vi "Autopatch.vi"() -> ()   [LabVIEW 2018]
uses:
  <vilib>/userdefined/High Color/IMAQdx.ctl
  <vilib>/DAQmx/write.llb/DAQmx Write (Analog DBL 1Chan 1Samp).vi
  <vilib>/DAQmx/write.llb/DAQmx Write (Analog Wfm 1Chan NSamp).vi
  <vilib>/DAQmx/read.llb/DAQmx Read (Analog Wfm 1Chan NSamp).vi
  <vilib>/Analysis/baseanly.llb/Mean (DBL).vi
  <vilib>/DAQmx/create/channels.llb/DAQmx Create Channel (AO-Voltage-Basic).vi
  <vilib>/DAQmx/miscellaneous.llb/DAQmx Fill In Error Info.vi
  <vilib>/DAQmx/create/channels.llb/DAQmx Create Channel (AI-Voltage-Basic).vi
  <vilib>/DAQmx/configure/timing.llb/DAQmx Timing (Sample Clock).vi
  <vilib>/DAQmx/configure/trigger.llb/DAQmx Start Trigger (Digital Edge).vi
  <vilib>/Waveform/WDTOps.llb/WDT Waveform Duration DBL.vi
  <vilib>/addons/control/pid/pid.llb/PID (DBL).vi
  <vilib>/vision/driver/NI_Vision_Acquisition_Software.lvlib
  <vilib>/addons/control/pid/NI_PID_pid.lvlib
  <vilib>/vision/NI_Vision_Development_Module.lvlib
  <vilib>/measure/NI_MABase.lvlib
  <vilib>/Analysis/NI_AALBase.lvlib
  <resource>/objmgr/daqmx.rc
panel:
  in  "下降步伐/um":dbl=1.0
  out "封接负压增幅":dbl
  out "气压波形图表":cluster{dbl, "低负":dbl}(graph)
  in  "case":dbl
  in  "低负开关":bool
  in  "低正开关":bool
  in  "大气压":bool
  in  "高负开关":bool
  in  "高正开关":bool
  in  "低负":sgl(knob)=-0.22290154
  in  "高负":sgl(knob)=-1.1416342
  in  "低正":sgl(knob)=0.7104824 scale=0.0..2.0
  in  "高正":sgl(knob)=15.0 scale=0.0..15.0
  out "给定值":dbl
  out "测量值":dbl
  out "错误输出 2":errorcluster caption="错误输出"
  in  "DevIndex":i32
  in  "采样率":u32=255
  out "循环时间":u32
  out "！":bool
  in  "自动破膜":bool
  in  "自动封接":bool
  in  "入液阻值校准":bool
  in  "阻值数组":dbl[](array[numeric])
  in  "针尖模板匹配":bool
  in  "自动接触":bool
  in  "文件路径（使用对话框）":path=path "E:/膜片/实验/数据"
  in  "保存图像和数据":bool
  in  "控制箱刺激/放大器刺激":bool=TRUE
  in  "frequency":dbl=20.0
  in  "Averaging":i32=3
  in  "amplitude":dbl=0.01
  in  "下拉列表":u16(ring) items=["Voltage Clamp", "Current Clamp"]
  in  "Holding Voltage":dbl
  out "Resistance":dbl
  out "电阻值2":dbl
  out "阻值波形图表":dbl(graph)
  out "校准的入液阻值":dbl
  in  "Session In":T1="cam1"
  out "目标坐标":i32[](array[numeric])
  in  "Number of Erosion":i32=10
  in  "Operation":T2(ring)=enum."Dilate"
  out "布尔":bool
  in  "自动聚焦":bool
  in  "细调焦":bool
  in  "Range":cluster{"Lower value":sgl, "Upper value":sgl}={"Lower value"=0.0, "Upper value"=86.0} {"Upper value" format="%.2f"; "Lower value" format="%.2f"}
  in  "Minimum Match Score":sgl=500.0 min=0 max=1000 format="%.2f"
  out "Number of Matches":i32
  in  "自动移动":bool
  out "Image":T3(plugin-control)
  in  "停止":bool
  out "错误输出":errorcluster
  in  "基路径":path=path "E:/膜片/膜片钳/程序/CCD/模板40倍.jpg"
  out "针尖坐标":sgl[](array[numeric])
  out "电信号波形图":waveform(dbl)(graph)
  out "Negative Peak":dbl
  out "mean":dbl caption="均值" format="%0.2f"
  in  "Minimum Contrast":i32 min=0 max=255 step=1
  in  "Number of Matches Requested":i32=1 min=1
  out "Matches 2":T4(array[cluster]) {"Bounding Box"."y" format="%.2f"; "Bounding Box"."x" format="%.2f"; "Position"."y" format="%.2f"; "Position"."x" format="%.2f"; "Score" format="%.2f"; "Scale" format="%.2f"; "Angle" format="%.2f"}
  in  "Match Mode":u16(ring) items=["Shift Invariant", "Rotation Invariant"]
  out "二值化":T3(plugin-control)
  in  "PID gains":T5={"proportional gain (Kc)"=-0.5, "integral time (Ti, min)"=0.0, "derivative time (Td, min)"=0.0} caption="PID增益" {"derivative time (Td, min)" format="%.3f"; "integral time (Ti, min)" format="%.3f"; "proportional gain (Kc)" format="%.3f"}
  in  "PID gains 2":T5={"proportional gain (Kc)"=0.5, "integral time (Ti, min)"=0.0, "derivative time (Td, min)"=0.0} caption="PID增益" {"derivative time (Td, min)" format="%.3f"; "integral time (Ti, min)" format="%.3f"; "proportional gain (Kc)" format="%.3f"}
  out "评价函数":dbl(graph)
  in  "聚焦值数组":dbl[](array[numeric])
  out "数组最大值":dbl
  out "调焦值2":dbl
  out "数值 3":dbl
  out "数值 4":dbl
  out "变量":dbl
  out "x+y 2":i16
  out "Particle Reports (Pixels)":T6(array[cluster]) {"Orientation" format="%.2f"; "Dimensions"."Height" format="%.2f"; "Dimensions"."Width" format="%.2f"; "Center of Mass"."Y" format="%.2f"; "Center of Mass"."X" format="%.2f"; "Bounding Rect"."Bottom" format="%.2f"; "Bounding Rect"."Right" format="%.2f"; "Bounding Rect"."Top" format="%.2f"; "Bounding Rect"."Left" format="%.2f"; "Number of Holes" format="%.2f"; "Area" format="%.2f"}
  out "Right":dbl
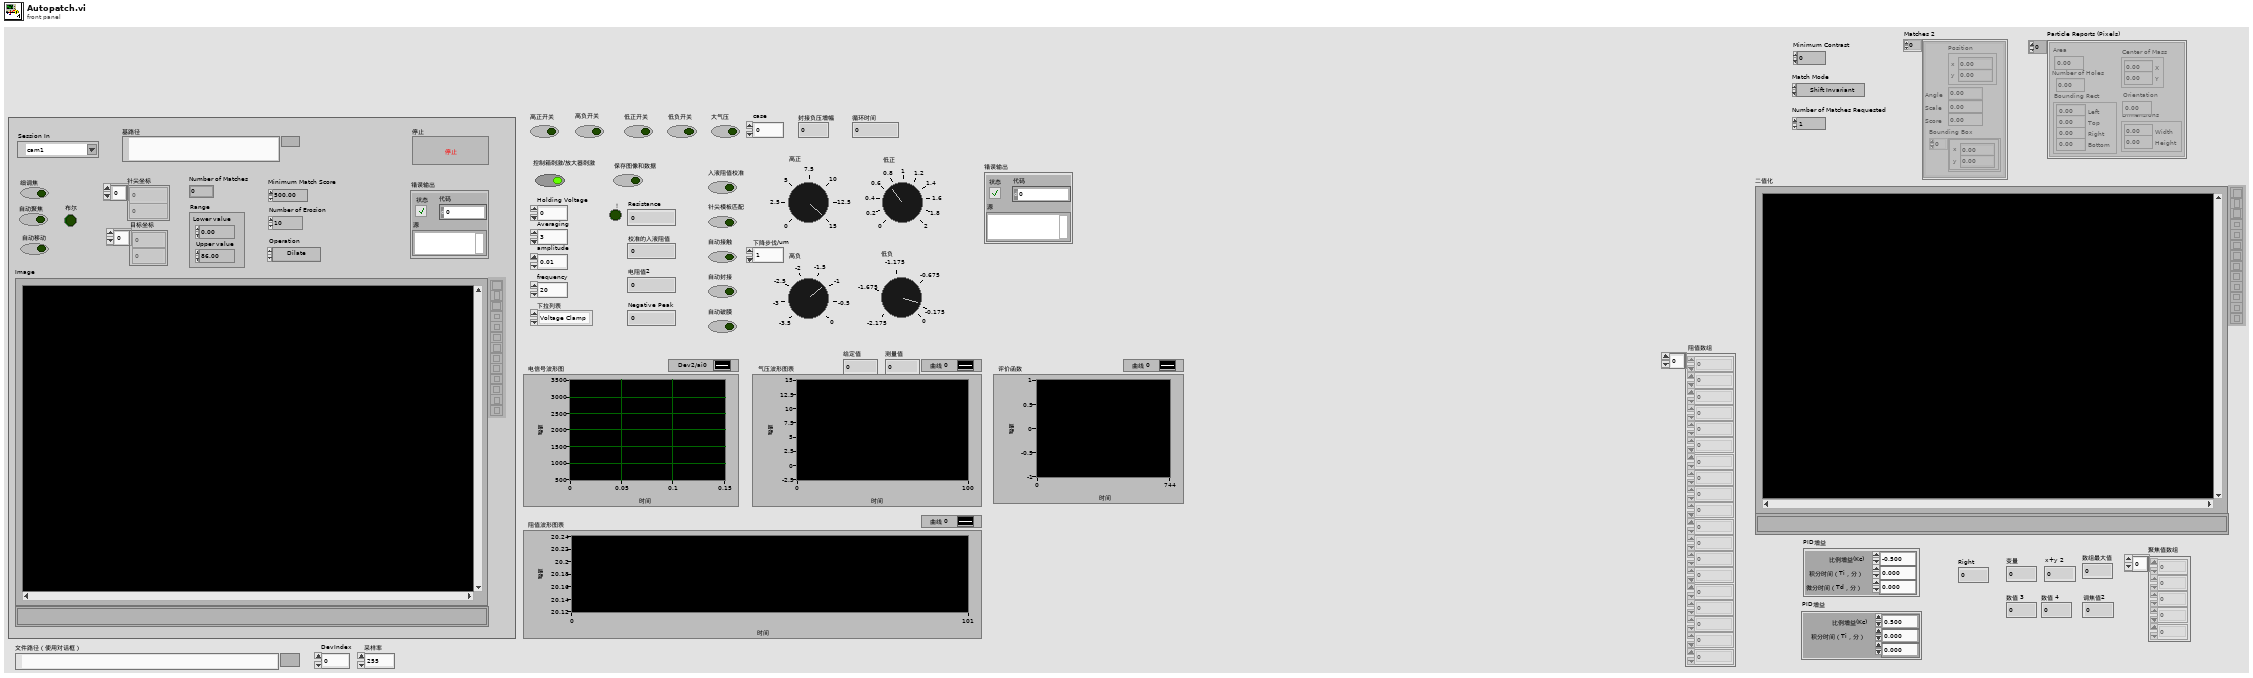
[diagram p1: front panel]
types:
  T1 = typedef "IMAQdx.ctl" = refnum<k21>
  T2 = enum32{"AutoM", "Close", "Dilate", "Erode", "Gradient", "Gradient out", "Gradient in", "Hit miss", "Open", "PClose", "POpen", "Thick", "Thin"}
  T3 = typedef "IMAQ Image.ctl" = refnum<image>
  T4 = cluster{"Position":cluster{"x":sgl, "y":sgl}, "Angle":sgl, "Scale":sgl, "Score":sgl, "Bounding Box":cluster{"x":sgl, "y":sgl}[]}[]
  T5 = cluster{"proportional gain (Kc)":dbl, "integral time (Ti, min)":dbl, "derivative time (Td, min)":dbl}
  T6 = cluster{"Area":dbl, "Number of Holes":dbl, "Bounding Rect":cluster{"Left":dbl, "Top":dbl, "Right":dbl, "Bottom":dbl}, "Center of Mass":cluster{"X":dbl, "Y":dbl}, "Orientation":dbl, "Dimensions":cluster{"Width":dbl, "Height":dbl}}[]
  T7 = typedef "Image Type" = u32
  T8 = enum16{"open", "replace", "create", "open or create", "replace or create", "replace or create with confirmation"}
  T9 = cluster{"Averaging":i32, "frequency":dbl, "amplitude":dbl, "Proportion":dbl, "Fs":dbl}
  T10 = enum16{"Sine Wave", "Triangle Wave", "Square Wave", "Sawtooth Wave"}
  T11 = cluster{"Position":cluster{"x":sgl, "y":sgl}, "Angle":sgl, "Scale":sgl, "Score":sgl, "Bounding Box":cluster{"x":sgl, "y":sgl}[]}
  T12 = cluster{"Global Rectangle":i32[], "Contours":cluster{"Contour Type":u32, "ROI Type":u32, "Points":i32[]}[]}
  T13 = cluster{"Area":dbl, "Number of Holes":dbl, "Bounding Rect":cluster{"Left":dbl, "Top":dbl, "Right":dbl, "Bottom":dbl}, "Center of Mass":cluster{"X":dbl, "Y":dbl}, "Orientation":dbl, "Dimensions":cluster{"Width":dbl, "Height":dbl}}
  T14 = cluster{"Left":dbl, "Top":dbl, "Right":dbl, "Bottom":dbl}
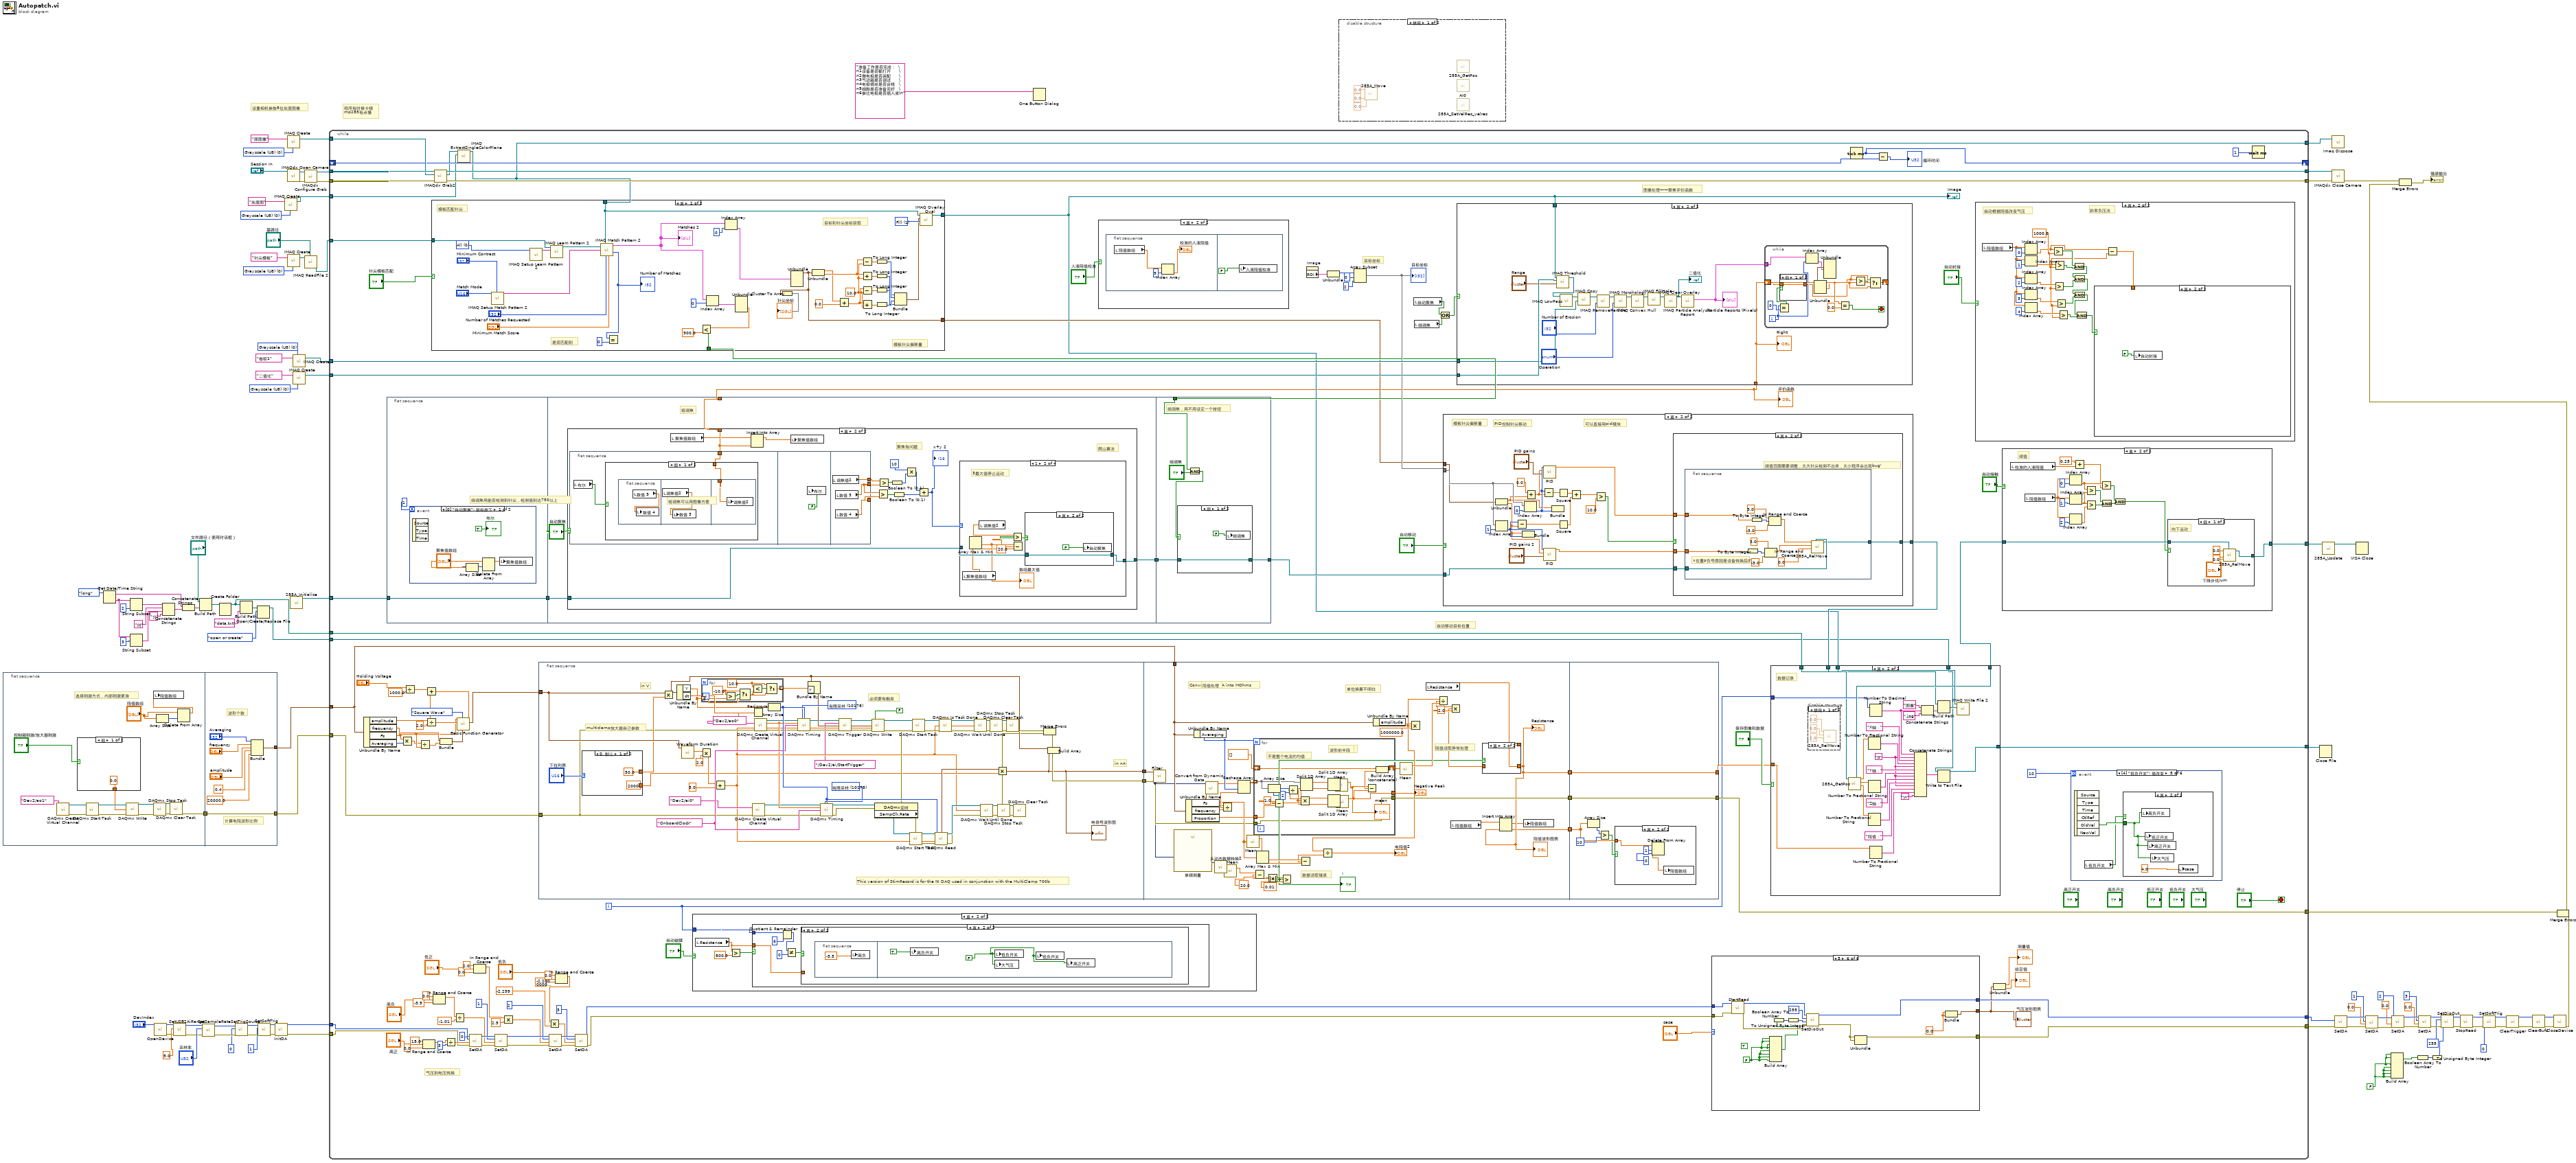
[diagram p0: block diagram]
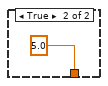
[diagram p2: hidden frame]
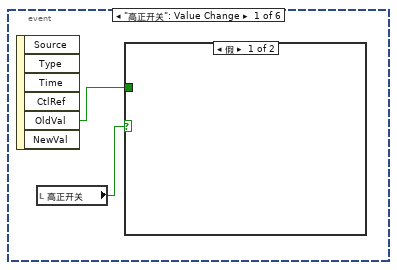
[diagram p4: hidden frame]
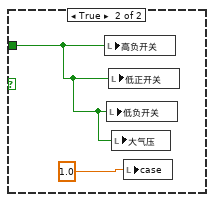
[diagram p5: hidden frame]
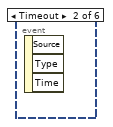
[diagram p6: hidden frame]
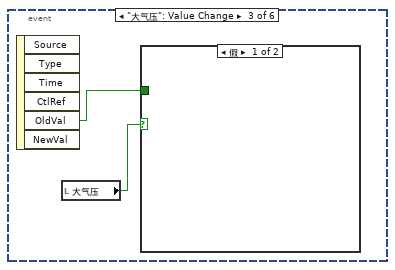
[diagram p7: hidden frame]
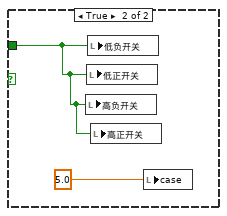
[diagram p8: hidden frame]
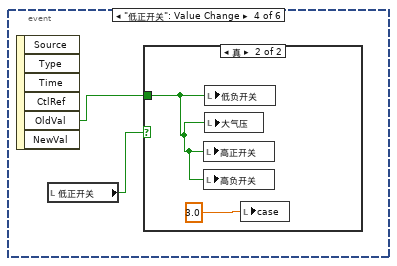
[diagram p9: hidden frame]
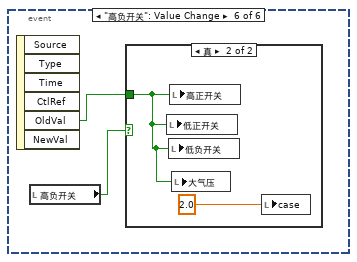
[diagram p12: hidden frame]
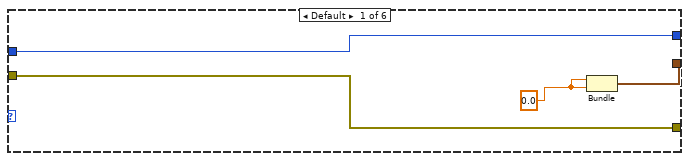
[diagram p14: hidden frame]
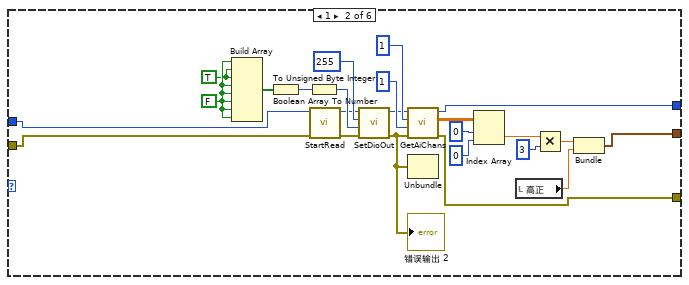
[diagram p15: hidden frame]
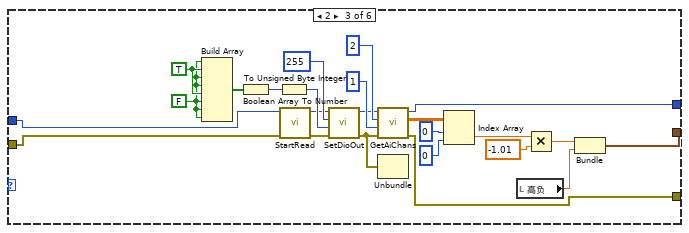
[diagram p16: hidden frame]
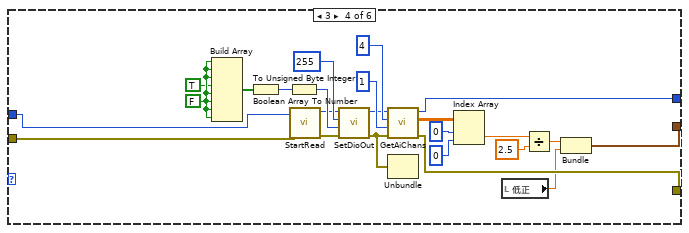
[diagram p17: hidden frame]
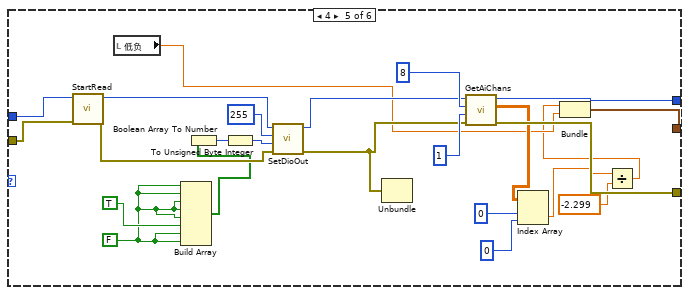
[diagram p18: hidden frame]
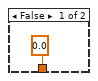
[diagram p19: hidden frame]
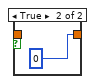
[diagram p20: hidden frame]
diagram:
  w12 = FALSE
  w55 = T7 0 items=["Grayscale (U8)", "Grayscale (I16)", "Grayscale (SGL)", "Complex (CSG)", "RGB (U32)", "HSL (U32)", "RGB (U64)", "Grayscale (U16)"] ("Image Type")
  w57 = T7 0 items=["Grayscale (U8)", "Grayscale (I16)", "Grayscale (SGL)", "Complex (CSG)", "RGB (U32)", "HSL (U32)", "RGB (U64)", "Grayscale (U16)"] ("Image Type")
  w58 = T7 0 items=["Grayscale (U8)", "Grayscale (I16)", "Grayscale (SGL)", "Complex (CSG)", "RGB (U32)", "HSL (U32)", "RGB (U64)", "Grayscale (U16)"] ("Image Type")
  w59 = T7 0 items=["Grayscale (U8)", "Grayscale (I16)", "Grayscale (SGL)", "Complex (CSG)", "RGB (U32)", "HSL (U32)", "RGB (U64)", "Grayscale (U16)"] ("Image Type")
  w60 = T7 0 items=["Grayscale (U8)", "Grayscale (I16)", "Grayscale (SGL)", "Complex (CSG)", "RGB (U32)", "HSL (U32)", "RGB (U64)", "Grayscale (U16)"] ("Image Type")
  # "程序有时候卡顿\nmp285有点慢"
  # "设置相机参数8位灰度图像"
  n1 = flat-sequence {
    tunnel: [w109] -> w62
    tunnel: [w124] -> w81
    tunnel: [w123] -> w61
    tunnel: w62 -> [w123]
    frame #0 {
      # "选择刺激方式，内部刺激更准"
      n2 = call-poly <vilib>:"DAQmx Create Virtual Channel.vi"("physical channels"=tag "Dev2/ao1") -> ("task out"=w116:refnum<k21>, "error out"=w115:errorcluster)  [unwired: 13 in]
      n3 = case shown="假" "控制箱刺激/放大器刺激" {
        tunnel: [0.0 ("data") 5.0 ("data")] -> w112
        frame False {
        }
        frame True {
        }
      }
      n4 = call <vilib>:"DAQmx Start Task.vi"("task/channels in"=w116, "error in"=w115) -> ("task out"=w117:refnum<k21>, "error out"=w118:errorcluster)  [unwired: 12 in]
      n5 = call-poly <vilib>:"DAQmx Write.vi"("task/channels in"=w117, "data"=w112, "error in"=w118) -> ("task out"=w119:refnum<k21>, "error out"=w120:errorcluster)  [unwired: 10 in, 1 out]
      n6 = call <vilib>:"DAQmx Stop Task.vi"("task/channels in"=w119, "error in"=w120) -> ("task out"=w113:refnum<k21>, "error out"=w114:errorcluster)  [unwired: 12 in]
      n7 = Array Size(array="阻值数组") -> (size(s)=w108:i32)
      n8 = call <vilib>:"DAQmx Clear Task.vi"("task in"=w113, "error in"=w114) -> ("error out"=w109:errorcluster)  [unwired: 13 in]
      n9 = Delete From Array(array="阻值数组", length=w108) -> (array with subset deleted=w106:dbl[])  [unwired: 1 in, 1 out]
      n10 = local write "阻值数组"(w106) -> ()
    }
    frame #1 {
      # "波形个数"
      # "计算电阻波形比例"
      n11 = Bundle("Averaging"="Averaging", "frequency"="frequency", "amplitude"="amplitude", "Proportion"=0.4, "Fs"=20000.0) -> (w124:T9)  [unwired: 1 in]
    }
  }
  n12 = Get Date/Time String(date format (0)=enum16{"short", "long", "abbreviated"}."long" ("日期格式(0)")) -> (date string=w77:string, time string=w73:string)  [unwired: 2 in]
  n13 = String Subset(string=w73, length (rest)=2 ("长度（剩余）")) -> (substring=w71:string)  [unwired: 1 in]
  n14 = String Subset(string=w73, offset (0)=3 ("偏移量(0)")) -> (substring=w69:string)  [unwired: 1 in]
  n15 = call "OpenDevice.vi"("DevIndex"="DevIndex") -> ("错误输出"=w39:errorcluster, "DevIndex Output"=w37:i32)  [unwired: 9 in]
  n16 = Concatenate Strings(w71, "时" ("字符串"), w69, "分" ("字符串")) -> (w70:string)
  n17 = call "SetUSB2AiRange.vi"("错误输入（无错误）"=w39, "Range"=sgl 5.0, "DevIndex"=w37) -> ("错误输出"=w48:errorcluster, "DevIndex Output"=w46:i32)  [unwired: 7 in]
  n18 = Concatenate Strings(w77, w70) -> (w66:string)
  n19 = Build Path(base path="文件路径（使用对话框）", name or relative path=w66) -> (appended path=w67:path)
  n20 = call "SetSampleRate.vi"("错误输入（无错误）"=w48, "SampleRate"="采样率", "DevIndex"=w46) -> ("错误输出"=w49:errorcluster, "DevIndex Output"=w47:i32)  [unwired: 7 in]
  n21 = Create Folder(path (use dialog)=w67) -> (created path=w65:path)  [unwired: 2 in, 2 out]
  n22 = call "SetTrigSource.vi"("错误输入（无错误）"=w49, "TrigSource"=u8 0, "DevIndex"=w47) -> ("错误输出"=w44:errorcluster, "DevIndex Output"=w43:i32)  [unwired: 7 in]
  n23 = Build Path(base path=w65, name or relative path="data.txt" ("字符串")) -> (appended path=w56:path)
  n24 = Open/Create/Replace File(file path (use dialog)=w56, operation (0:open)=T8."open or create" ("操作(0:open)")) -> (refnum out=w52:refnum<file>)  [unwired: 4 in, 2 out]
  n25 = call "SetSoftTrig.vi"("错误输入（无错误）"=w44, "Trig"=u8 1, "DevIndex"=w43) -> ("错误输出"=w40:errorcluster, "DevIndex Output"=w38:i32)  [unwired: 7 in]
  n26 = call "InitDA.vi"("错误输入（无错误）"=w40, "DevIndex"=w38) -> ("错误输出"=w34:errorcluster, "DevIndex Output"=w35:i32)  [unwired: 8 in]
  n27 = call "IMAQ Create"("Image Name"="灰度图", "Image Type"=w55) -> ("New Image"=w53:T3)  [unwired: 3 in, 1 out]
  n28 = call "IMAQ Create"("Image Name"="原图像", "Image Type"=w60) -> ("New Image"=w95:T3)  [unwired: 3 in, 1 out]
  n29 = call <vilib>:"IMAQdx Open Camera.vi"("Session In"="Session In") -> ("error out"=w104:errorcluster, "Session Out"=w103:T1)  [unwired: 9 in]
  n30 = call "IMAQ Create"("Image Name"="针尖模板", "Image Type"=w59) -> ("New Image"=w90:T3)  [unwired: 3 in, 1 out]
  n31 = call "285A_Initialize.vi"() -> ("VISA资源名称输出"=w82:refnum<visa-resource-name>)  [unwired: 10 in, 1 out]
  n32 = call "IMAQ Create"("Image Name"="卷积1", "Image Type"=w58) -> ("New Image"=w87:T3)  [unwired: 3 in, 1 out]
  n33 = call "IMAQ Create"("Image Name"="二值化", "Image Type"=w57) -> ("New Image"=w86:T3)  [unwired: 3 in, 1 out]
  n34 = call <vilib>:"IMAQdx Configure Grab.vi"("error in"=w104, "Session In"=w103) -> ("error out"=w102:errorcluster, "Session Out"=w101:T1)  [unwired: 8 in]
  n35 = call "IMAQ ReadFile 2"("File Path"="基路径", "Image"=w90) -> ("Image Out"=w89:T3)  [unwired: 5 in, 4 out]
  n36 = while {
    tunnel: w101 -> [w244]
    tunnel: w95 -> [w243]
    tunnel: [w242] -> w96
    tunnel: [w185] -> w97
    tunnel: w102 -> [w240]
    tunnel: [w239] -> w98
    tunnel: w89 -> [w238]
    tunnel: w87 -> [w233]
    tunnel: w86 -> [w237]
    tunnel: w82 -> [w234]
    tunnel: [w193] -> w84
    tunnel: w81 -> [w148]
    tunnel: w61 -> [w213]
    tunnel: [w198] -> w79
    tunnel: w65 -> [w207]
    shift-right: [w188] -> _
    shift-left: _ -> [w189]
    tunnel: w53 -> [w184]
    tunnel: w52 -> [w179]
    tunnel: [w178] -> w51
    tunnel: w35 -> [w160]
    tunnel: w34 -> [w159]
    tunnel: [w153] -> w3
    tunnel: [w156] -> w2
    i -> [w147]
    stop <- "停止" stop-if-true
    # "气压到电压转换"
    # "目标坐标"
    # "图像处理——聚焦评价函数"
    # "自动移动目标位置"
    # "粗调焦可以用图像方差"
    # "细调焦用能否检测到针尖，检测值到达750以上"
    n37 = Unbundle By Name(w148) -> ("amplitude"=w218:dbl, "frequency"=w217:dbl, "Fs"=w219:dbl, "Averaging"=w220:i32)
    n38 = flat-sequence {
      tunnel: w234 -> [w716]
      tunnel: [w716] -> w236
      tunnel: w236 -> [w723]
      tunnel: [w722] -> w235
      tunnel: w180 -> [w721]
      tunnel: [w803] -> w232
      tunnel: w235 -> [w804]
      tunnel: w229 -> [w801]
      frame #0 {
        n39 = event shown="[0] \"自动聚焦\": 鼠标按下" {
          selector: _ -> [_ _]
          dyn-events: _ -> [_ _]
          timeout: 1 -> [_ _]
          event "自动聚焦": Mouse Down {
            n40 = event-data() -> ()  [unwired: 1 in, 3 out]
            n41 = Array Size(array="聚焦值数组") -> (size(s)=w717:i32)
            n42 = Delete From Array(array="聚焦值数组", length=w717) -> (array with subset deleted=w718:dbl[])  [unwired: 1 in, 1 out]
            n43 = local write "聚焦值数组"(w718) -> ()
            "布尔" <- TRUE
          }
          event Timeout {
            n44 = event-data() -> ()  [unwired: 1 in, 3 out]
          }
        }
      }
      frame #1 {
        # "粗调焦"
        n45 = case shown="真" "自动聚焦" {
          tunnel: w723 -> [w725 w734]
          tunnel: [w725 w733] -> w722
          tunnel: w721 -> [_ w732]
          frame False {
          }
          frame True {
            # "聚焦有问题"
            # "爬山算法"
            n46 = flat-sequence {
              tunnel: w732 -> [w742]
              tunnel: [w752] -> w740
              tunnel: [w751] -> w738
              tunnel: [w750] -> w739
              frame #0 {
                n47 = local read "布尔"() -> (w741:bool)
                n48 = case shown="假" w741 {
                  tunnel: w742 -> [w743 w747]
                  frame False {
                    n49 = flat-sequence {
                      tunnel: w743 -> [w746]
                      frame #0 {
                        n50 = local read "数值 3"() -> (w744:dbl)
                        n51 = local write "数值 4"(w744) -> ()
                      }
                      frame #1 {
                        n52 = local read "调焦值2"() -> (w745:dbl)
                        n53 = local write "数值 3"(w745) -> ()
                      }
                      frame #2 {
                        n54 = local write "调焦值2"(w746) -> ()
                      }
                    }
                  }
                  frame True {
                    # "第一次赋值"
                    "调焦值2" <- w747
                    "数值 3" <- w747
                    "数值 4" <- w747
                    "变量" <- 1
                  }
                }
              }
              frame #1 {
                n55 = local write "布尔"(FALSE) -> ()
              }
              frame #2 {
                n56 = local read "调焦值2"() -> (w752:dbl)
                n57 = local read "数值 3"() -> (w751:dbl)
                n58 = local read "数值 4"() -> (w750:dbl)
              }
            }
            n59 = local read "聚焦值数组"() -> (w731:dbl[])
            n60 = Insert Into Array(array=w731, new element=w732) -> (w730:dbl[])  [unwired: 1 in]
            n61 = local write "聚焦值数组"(w730) -> ()
            n62 = Greater?(x=w738, y=w739) -> (0:w737:bool)
            n63 = Greater?(x=w740, y=w738) -> (0:w729:bool)
            n64 = Boolean To (0,1)(Boolean=w729) -> (0, 1=w728:i16)
            n65 = Boolean To (0,1)(Boolean=w737) -> (0, 1=w727:i16)
            n66 = Multiply(x=i16 10, y=w728) -> (x*y=w735:i16)
            n67 = Add(x=w735, y=w727) -> (x+y=w726:i16)
            "x+y 2" <- w726
            n68 = case shown="1" w726 {
              tunnel: [w759 w764 w778 w786] -> w733
              tunnel: w734 -> [w757 w765 w777 w787]
              frame 11, Default {
                # "1往上运动"
                n69 = local read "变量"() -> (w753:dbl)
                n70 = Multiply(x=10.0 ("Z 2"), y=w753) -> (x*y=w754:dbl)
                n71 = call "285A_RelMove.vi"("VISA资源名称"=w757, "Z 2"=w754, "Y 2"=0.0, "X 2"=0.0) -> ("VISA resource name out 2"=w759:refnum<visa-resource-name>)  [unwired: 2 in, 5 out]
              }
              frame 1 {
                # "3最大值停止运动"
                n72 = local read "聚焦值数组"() -> (w760:dbl[])
                n73 = Array Max & Min(array=w760) -> (max value=w763:dbl)  [unwired: 3 out]
                "数组最大值" <- w763
                n74 = local read "调焦值2"() -> (w767:dbl)
                n75 = Subtract(x=w763, y=20.0) -> (x-y=w761:dbl)
                n76 = Greater?(x=w767, y=w761) -> (0:w766:bool)
                n77 = case shown="真" w766 {
                  tunnel: [w768 w775] -> w764
                  tunnel: w765 -> [w773 w775]
                  frame False {
                    n78 = local read "变量"() -> (w770:dbl)
                    n79 = Multiply(x=20.0 ("Z 2"), y=w770) -> (x*y=w771:dbl)
                    n80 = call "285A_RelMove.vi"("VISA资源名称"=w773, "Z 2"=w771, "Y 2"=0.0, "X 2"=0.0) -> ("VISA resource name out 2"=w768:refnum<visa-resource-name>)  [unwired: 2 in, 5 out]
                  }
                  frame True {
                    n81 = local write "自动聚焦"(FALSE) -> ()
                  }
                }
              }
              frame 10 {
                # "4继续向上运动"
                n82 = flat-sequence {
                  tunnel: [w783] -> w778
                  tunnel: w777 -> [w782]
                  frame #0 {
                    n83 = local read "变量"() -> (w779:dbl)
                    n84 = Multiply(x=10.0 ("Z 2"), y=w779) -> (x*y=w780:dbl)
                    n85 = call "285A_RelMove.vi"("VISA资源名称"=w782, "Z 2"=w780, "Y 2"=0.0, "X 2"=0.0) -> ("VISA resource name out 2"=w783:refnum<visa-resource-name>)  [unwired: 2 in, 5 out]
                  }
                }
              }
              frame 0 {
                # "2向回运动"
                n86 = flat-sequence {
                  tunnel: w787 -> [w792]
                  tunnel: [w792] -> w788
                  tunnel: [w797] -> w786
                  tunnel: w788 -> [w796]
                  frame #0 {
                    n87 = local read "变量"() -> (w791:dbl)
                    n88 = Multiply(x=w791, y=-1) -> (x*y=w789:dbl)
                    n89 = local write "变量"(w789) -> ()
                  }
                  frame #1 {
                    n90 = local read "变量"() -> (w793:dbl)
                    n91 = Multiply(x=10.0 ("Z 2"), y=w793) -> (x*y=w794:dbl)
                    n92 = call "285A_RelMove.vi"("VISA资源名称"=w796, "Z 2"=w794, "Y 2"=0.0, "X 2"=0.0) -> ("VISA resource name out 2"=w797:refnum<visa-resource-name>)  [unwired: 2 in, 5 out]
                  }
                }
              }
            }
          }
        }
      }
      frame #2 {
        # "细调焦，用不用设定一个按钮"
        n93 = And(x=w801, y="细调焦") -> (x .and. y?=w802:bool)
        n94 = case shown="假" w802 {
          tunnel: [w806 w807] -> w803
          tunnel: w804 -> [w806 w808]
          frame False {
            n95 = local write "细调焦"(FALSE) -> ()
          }
          frame True {
            n96 = local read "变量"() -> (w810:dbl)
            n97 = Multiply(x=10.0 ("Z 2"), y=w810) -> (x*y=w809:dbl)
            n98 = call "285A_RelMove.vi"("VISA资源名称"=w808, "Z 2"=w809, "Y 2"=0.0, "X 2"=0.0) -> ("VISA resource name out 2"=w807:refnum<visa-resource-name>)  [unwired: 2 in, 5 out]
          }
        }
      }
    }
    n99 = Multiply(x=w219, y=w220) -> (x*y=w215:dbl)
    n100 = Divide(x="Holding Voltage", y=1000.0) -> (x/y=w224:dbl)
    n101 = Divide(x=w215, y=w217) -> (x/y=w216:dbl)
    n102 = In Range and Coerce(upper limit=sgl 15.0 ("上限"), x="高正", lower limit=sgl 0.0 ("下限")) -> (coerced(x)=w132:sgl)  [unwired: 1 out]
    n103 = Divide(x=w218, y=2.0) -> (x/y=w223:dbl)
    n104 = Add(x=w224, y=w223) -> (x+y=w222:dbl)
    n105 = In Range and Coerce(upper limit=sgl 0.0 ("上限"), x="高负", lower limit=sgl -3.5 ("下限")) -> (coerced(x)=w136:sgl)  [unwired: 1 out]
    n106 = call <vilib>:"IMAQdx Grab2.vi"("error in"=w240, "Image In"=w243, "Session In"=w244) -> ("error out"=w239:errorcluster, "Image Out"=w186:T3, "Session Out"=w242:T1)  [unwired: 5 in, 1 out]
    n107 = Bundle("Fs"=w219, w216) -> (w221:cluster{"Fs":dbl, dbl})  [unwired: 1 in]
    n108 = Divide(x=w132, y=3) -> (x/y=w167:sgl)
    n109 = Divide(x=w136, y=-1.01) -> (x/y=w163:dbl)
    n110 = call <vilib>:"Basic Function Generator.vi"("offset"=w222, "sampling info"=w221, "signal type"=T10."Square Wave", "amplitude"=w223, "frequency"=w217) -> ("signal out"=w228:waveform(dbl))  [unwired: 4 in, 2 out]
    n111 = call "IMAQ ExtractSingleColorPlane"("Image Dst"=w184, "Image Src"=w186) -> ("Image Dst Out"=w185:T3)  [unwired: 8 in, 1 out]
    n112 = case shown="真" "针尖模板匹配" {
      tunnel: w238 -> [_ w519]
      tunnel: w185 -> [w479 w483]
      tunnel: [FALSE w518] -> w229
      tunnel: [w478 w486] -> w200
      tunnel: [w479 w482] -> w199
      frame False {
        w480 = 0.0 ("x")
        n113 = Bundle("x"=w480, "x"=w480) -> (w478:cluster{"x":dbl, "x":dbl})  [unwired: 1 in]
      }
      frame True {
        w485 = u32 1 items=["Frame", "Fill", "Highlight"] ("Drawing Mode (Frame)")
        w488 = 10.0 ("y")
        w512 = u16 0 items=["All", "Shift Information", "Rotation Information"] ("Learn Mode")
        # "目标和针尖坐标获取"
        # "模板针尖偏移量"
        # "是否匹配到"
        # "模板匹配针尖"
        n114 = call "IMAQ Setup Match Pattern 2"("Minimum Contrast"="Minimum Contrast", "Match Mode"="Match Mode") -> ("Match Pattern Setup Data"=w516:string)  [unwired: 8 in, 1 out]
        n115 = call "IMAQ Setup Learn Pattern 2"("Learn Mode"=w512) -> ("Learn Pattern Setup Data"=w511:string)  [unwired: 9 in, 1 out]
        n116 = call "IMAQ Learn Pattern 2"("Learn Pattern Setup Data"=w511, "Image"=w519) -> ("Template Image Out"=w508:T3)  [unwired: 8 in, 1 out]
        n117 = call "IMAQ Match Pattern 2"("Minimum Match Score"="Minimum Match Score", "Number of Matches Requested"="Number of Matches Requested", "Match Pattern Setup Data"=w516, "Template Image"=w508, "Image"=w483) -> ("Number of Matches"=w509:i32, "Matches"=w505:T4)  [unwired: 4 in, 1 out]
        "Number of Matches" <- w509
        "Matches 2" <- w505
        n118 = Equal?(x=w509, y=0) -> ()  [unwired: 1 out]
        n119 = Index Array(array=w505, index=0 ("索引")) -> (element=w503:T11)
        n120 = Index Array(array=w505, index=0 ("索引")) -> (element=w487:T11)
        n121 = Unbundle(w503) -> ("Score"=w502:sgl)  [unwired: 4 out]
        n122 = Less?(x=w502, y=sgl 900.0) -> (x < y?=w518:bool)
        n123 = Unbundle(w487) -> ("Position"=w486:cluster{"x":sgl, "y":sgl})  [unwired: 4 out]
        n124 = Cluster To Array(cluster=w486) -> (array=→"针尖坐标":sgl[])
        n125 = Unbundle(w486) -> ("x"=w497:sgl, "y"=w500:sgl)
        n126 = Add(x=w497, y=sgl 0.0) -> (x+y=w499:sgl)
        n127 = Subtract(x=w500, y=w488) -> (x-y=w491:dbl)
        n128 = Add(x=w500, y=w488) -> (x+y=w490:dbl)
        n129 = Subtract(x=w499, y=w488) -> (x-y=w489:dbl)
        n130 = Add(x=w499, y=w488) -> (x+y=w492:dbl)
        n131 = To Long Integer(number=w491) -> (32bit integer=w494:i32)
        n132 = To Long Integer(number=w490) -> (32bit integer=w495:i32)
        n133 = To Long Integer(number=w489) -> (32bit integer=w493:i32)
        n134 = To Long Integer(number=w492) -> (32bit integer=w496:i32)
        n135 = Bundle(w493, w494, w496, w495) -> (w484:cluster{i32, i32, i32, i32})  [unwired: 1 in]
        n136 = call "IMAQ Overlay Oval"("Drawing Mode (Frame)"=w485, "Bounding Rectangle"=w484, "Image"=w483) -> ("Image Out"=w482:T3)  [unwired: 7 in, 1 out]
      }
    }
    "Image" <- w199
    n137 = call "SetDA.vi"("错误输入（无错误）"=w159, "DAVolt"=w167, "DANum"=u8 0, "DevIndex"=w160) -> ("错误输出"=w176:errorcluster, "DevIndex Output"=w177:i32)  [unwired: 6 in]
    n138 = In Range and Coerce(upper limit=sgl 2.0 ("上限"), x="低正", lower limit=sgl 0.0 ("下限")) -> (coerced(x)=w140:sgl)  [unwired: 1 out]
    n139 = call "SetDA.vi"("错误输入（无错误）"=w176, "DAVolt"=w163, "DANum"=u8 1, "DevIndex"=w177) -> ("错误输出"=w175:errorcluster, "DevIndex Output"=w174:i32)  [unwired: 6 in]
    n140 = Multiply(x=w140, y=2.5) -> (x*y=w154:dbl)
    n141 = flat-sequence {
      tunnel: w228 -> [w596]
      tunnel: w213 -> [w592]
      tunnel: [w597] -> w212
      tunnel: [w581] -> w211
      tunnel: w212 -> [w665]
      tunnel: w211 -> [w666]
      tunnel: w148 -> [w667]
      tunnel: [w664] -> w197
      tunnel: [w654] -> w196
      tunnel: [w652] -> w195
      tunnel: [w709] -> w208
      tunnel: [w710] -> w198
      tunnel: w197 -> [w710]
      tunnel: w196 -> [w709]
      tunnel: w195 -> [w707]
      frame #0 {
        w626 = 10178 items=["有限采样"=10178, "连续采样"=10123, "硬件定时单点"=12522] ("sample mode")
        w627 = tag "OnboardClock" ("source")
        w619 = 10178 items=["有限采样"=10178, "连续采样"=10123, "硬件定时单点"=12522] ("sample mode")
        # "必须要有触发"
        # "This version of StimRecord is for the NI DAQ used in conjunction with the MultiClamp 700b"
        # "multiclamp放大器自己参数"
        # "in V"
        # "in nA"
        n142 = case shown="0, 默认" "下拉列表" {
          tunnel: [50.0 ("y") 2500000000.0 ("y")] -> w593
          tunnel: [2000.0 ("y") 0.1 ("y")] -> w594
          frame 0, Default {
          }
          frame 1 {
          }
        }
        n143 = Multiply(x=w596, y=w593) -> (x*y=w612:waveform(dbl))
        n144 = Unbundle By Name(w612) -> ("Y"=w580:dbl[], "dt"=w611:dbl)
        n145 = call-poly <vilib>:"Waveform Duration.vi"("waveform in"=w596) -> ("duration"=w614:dbl)  [unwired: 8 in, 2 out]
        n146 = Multiply(x=w614, y=2.0) -> (x*y=w615:dbl)
        n147 = for {
          tunnel: [w641] -> w579 mode=indexing
          tunnel: w580 -> [w635] mode=indexing
          w636 = 10.0 ("t")
          w639 = -10.0 ("t")
          n148 = Greater?(x=w639, y=w635) -> (0:w640:bool)
          n149 = Select(t=w639, s=w640, f=w635) -> (s? t:f=w637:dbl)
          n150 = Less?(x=w636, y=w637) -> (x < y?=w638:bool)
          n151 = Select(t=w636, s=w638, f=w637) -> (s? t:f=w641:dbl)
        }
        n152 = Add(x=w615, y=5.0) -> (x+y=w583:dbl)
        n153 = Reciprocal(x=w611) -> (1/x=w620:dbl)
        n154 = call-poly <vilib>:"DAQmx Create Virtual Channel.vi"("physical channels"=tag "Dev2/ai0", "error in"=w592) -> ("task out"=w618:refnum<k21>, "error out"=w617:errorcluster)  [unwired: 12 in]
        n155 = call-poly <vilib>:"DAQmx Create Virtual Channel.vi"("physical channels"=tag "Dev2/ao0", "error in"=w592) -> ("task out"=w607:refnum<k21>, "error out"=w606:errorcluster)  [unwired: 12 in]
        n156 = Array Size(array=w580) -> (size(s)=w634:i32)
        n157 = call-poly <vilib>:"DAQmx Timing.vi"("task/channels in"=w607, "sample mode"=w626, "samples per channel"=w634, "rate"=w620, "source"=w627, "error in"=w606) -> ("task out"=w591:refnum<k21>, "error out"=w589:errorcluster)  [unwired: 8 in]
        n158 = Bundle By Name(cluster=w612, "Y"=w579) -> (w613:waveform(dbl))
        n159 = call-poly <vilib>:"DAQmx Timing.vi"("task/channels in"=w618, "sample mode"=w619, "samples per channel"=w634, "rate"=w620, "source"=w627, "error in"=w617) -> ("task out"=w622:refnum<k21>, "error out"=w623:errorcluster)  [unwired: 8 in]
        n160 = call-poly <vilib>:"DAQmx Trigger.vi"("task/channels in"=w591, "source"=tag "/Dev2/ai/StartTrigger", "error in"=w589) -> ("task out"=w590:refnum<k21>, "error out"=w588:errorcluster)  [unwired: 11 in]
        n161 = call-poly <vilib>:"DAQmx Write.vi"("task/channels in"=w590, "auto start"=FALSE, "data"=w613, "timeout"=w583, "error in"=w588) -> ("task out"=w610:refnum<k21>, "error out"=w631:errorcluster)  [unwired: 8 in, 1 out]
        n162 = property class="DAQmx定时" props=["SampClk.Rate"](reference=w622, error in=w623) -> (reference out=w624:refnum<k21>)  [unwired: 2 out]
        n163 = call <vilib>:"DAQmx Start Task.vi"("task/channels in"=w610, "error in"=w631) -> ("task out"=w628:refnum<k21>, "error out"=w630:errorcluster)  [unwired: 12 in]
        n164 = call <vilib>:"DAQmx Start Task.vi"("task/channels in"=w624, "error in"=w630) -> ("task out"=w602:refnum<k21>, "error out"=w603:errorcluster)  [unwired: 12 in]
        n165 = call-poly <vilib>:"DAQmx Read.vi"("task/channels in"=w602, "number of samples per channel"=w634, "timeout"=w583, "error in"=w603) -> ("task out"=w587:refnum<k21>, "data"=w616:waveform(dbl), "error out"=w585:errorcluster)  [unwired: 9 in]
        n166 = call <vilib>:"DAQmx Is Task Done.vi"("task/channels in"=w628, "error in"=w630) -> ("task out"=w629:refnum<k21>, "error out"=w632:errorcluster)  [unwired: 11 in, 1 out]
        n167 = call <vilib>:"DAQmx Wait Until Done.vi"("task/channels in"=w629, "timeout (sec)"=w583, "error in"=w632) -> ("task out"=w608:refnum<k21>, "error out"=w609:errorcluster)  [unwired: 11 in]
        n168 = call <vilib>:"DAQmx Wait Until Done.vi"("task/channels in"=w587, "timeout (sec)"=w583, "error in"=w585) -> ("task out"=w586:refnum<k21>, "error out"=w584:errorcluster)  [unwired: 11 in]
        n169 = call <vilib>:"DAQmx Stop Task.vi"("task/channels in"=w608, "error in"=w609) -> ("task out"=w605:refnum<k21>, "error out"=w604:errorcluster)  [unwired: 12 in]
        n170 = Multiply(x=w616, y=w594) -> (x*y=w581:waveform(dbl))
        "电信号波形图" <- w581
        n171 = call <vilib>:"DAQmx Stop Task.vi"("task/channels in"=w586, "error in"=w584) -> ("task out"=w600:refnum<k21>, "error out"=w601:errorcluster)  [unwired: 12 in]
        n172 = call <vilib>:"DAQmx Clear Task.vi"("task in"=w605, "error in"=w604) -> ("error out"=w633:errorcluster)  [unwired: 13 in]
        n173 = call <vilib>:"DAQmx Clear Task.vi"("task in"=w600, "error in"=w601) -> ("error out"=w599:errorcluster)  [unwired: 13 in]
        n174 = Merge Errors(w633, w599) -> (w597:errorcluster)
        n175 = Build Array(w612, w581) -> ()  [unwired: 1 out]
      }
      frame #1 {
        # "数据读取错误"
        # "阻值读取异常处理"
        # "单位换算不明白"
        # "阻值处理"
        # "Convert Volts/pA into MOhms"
        n176 = call "Filter"("error in (no error)"=w665, "Signal"=w666) -> ("error out"=w668:errorcluster, "Filtered Signal"=w657:dynamicdata)  [unwired: 8 in]
        n177 = call "单频测量"("Signals"=w657) -> ("Frequency"=w656:dynamicdata)  [unwired: 9 in, 1 out]
        n178 = Unbundle By Name(w667) -> ("Fs"=w681:dbl, "frequency"=w680:dbl, "Proportion"=w673:dbl)
        n179 = Unbundle By Name(w667) -> ("Averaging"=w679:i32)
        n180 = call "Convert from Dynamic Data"("Dynamic Data Type"=w657) -> ("Array"=w671:dbl[])  [unwired: 3 in]
        n181 = call "从动态数据转换2"("Dynamic Data Type"=w656) -> ("Array"=w655:dbl[])  [unwired: 3 in]
        n182 = Divide(x=w681, y=w680) -> (x/y=w684:dbl)
        n183 = call-poly <vilib>:"Mean.vi"("X"=w655) -> ("mean"=w651:dbl)  [unwired: 1 out]
        n184 = Reshape Array(w671, w679, w684) -> (w683:dbl[][])
        n185 = call-poly <vilib>:"Mean.vi"("X"=w671) -> ("mean"=w672:dbl)  [unwired: 1 out]
        n186 = Subtract(x=w651, y=sgl 20.0) -> (x-y=w649:dbl)
        n187 = for {
          N: w679 -> [_]
          tunnel: w683 -> [w695] mode=indexing
          tunnel: w668 -> [w702]
          shift-right: [w703] -> w682
          shift-left: dbl[] [] -> [w704]
          tunnel: [w690] -> w678
          tunnel: [w702] -> w664
          tunnel: w673 -> [w694]
          # "不是整个电流的均值"
          # "波形后半段"
          # "波形前半段"
          n188 = Array Size(array=w695) -> (size(s)=w692:i32)
          n189 = Subtract(x=1.0, y=w694) -> (x-y=w697:dbl)
          n190 = Divide(x=w692, y=2) -> (x/y=w699:dbl)
          n191 = Multiply(x=w699, y=w697) -> (x*y=w696:dbl)
          n192 = Split 1D Array(array=w695, index=w699) -> (first subarray=w691:dbl[], second subarray=w700:dbl[])
          n193 = Split 1D Array(array=w691, index=w696) -> (second subarray=w687:dbl[])  [unwired: 1 out]
          n194 = Split 1D Array(array=w700, index=w696) -> (second subarray=w688:dbl[])  [unwired: 1 out]
          n195 = call-poly <vilib>:"Mean.vi"("X"=w687) -> ("mean"=w689:dbl)  [unwired: 1 out]
          "mean" <- w689
          n196 = call-poly <vilib>:"Mean.vi"("X"=w688) -> ("mean"=w690:dbl)  [unwired: 1 out]
          n197 = Subtract(x=w689, y=w690) -> (x-y=w693:dbl)
          n198 = Build Array (concatenate)(w704, w693) -> (w703:dbl[])
        }
        "Negative Peak" <- w678
        n199 = Array Max & Min(array=w671) -> (min value=w670:dbl)  [unwired: 3 out]
        n200 = Absolute Value(x=w649) -> (abs(x)=w648:dbl)
        n201 = Greater?(x=w648, y=0.01) -> (0:w646:bool)
        "！" <- w646
        n202 = Subtract(x=w672, y=w670) -> (x-y=w669:dbl)
        n203 = Unbundle By Name(w667) -> ("amplitude"=w676:dbl)
        n204 = call-poly <vilib>:"Mean.vi"("X"=w682) -> ("mean"=w677:dbl)  [unwired: 1 out]
        n205 = Multiply(x=w676, y=1000000.0) -> (x*y=w662:dbl)
        n206 = Divide(x=w662, y=w669) -> (x/y=→"电阻值2":dbl)
        n207 = local read "Resistance"() -> (w659:dbl)
        n208 = Divide(x=w662, y=w677) -> (x/y=w660:dbl)
        n209 = Multiply(x=w660, y=2.0) -> (x*y=w658:dbl)
        n210 = local read "阻值数组"() -> (w653:dbl[])
        n211 = case shown="真" w646 {
          tunnel: w659 -> [_ w686]
          tunnel: w658 -> [w685 _]
          tunnel: [w685 w686] -> w654
          frame False {
          }
          frame True {
          }
        }
        "阻值波形图表" <- w654
        "Resistance" <- w654
        n212 = Insert Into Array(array=w653, new element=w654) -> (w652:dbl[])  [unwired: 1 in]
        n213 = local write "阻值数组"(w652) -> ()
      }
      frame #2 {
        n214 = Array Size(array=w707) -> (size(s)=w706:i32)
        n215 = Greater?(x=w706, y=10) -> (0:w705:bool)
        n216 = case shown="真" w705 {
          tunnel: w707 -> [_ w714]
          frame False {
          }
          frame True {
            n217 = Delete From Array(array=w714, length=1 ("长度"), index=0 ("索引")) -> (array with subset deleted=w711:dbl[])  [unwired: 1 out]
            n218 = local write "阻值数组"(w711) -> ()
          }
        }
      }
    }
    n219 = call "SetDA.vi"("错误输入（无错误）"=w175, "DAVolt"=w154, "DANum"=u8 2, "DevIndex"=w174) -> ("错误输出"=w172:errorcluster, "DevIndex Output"=w173:i32)  [unwired: 6 in]
    n220 = In Range and Coerce(upper limit=sgl 0.0 ("上限"), x="低负", lower limit=sgl -2.2 ("下限")) -> (coerced(x)=w142:sgl)  [unwired: 1 out]
    n221 = Multiply(x=w142, y=-2.299) -> (x*y=w161:dbl)
    n222 = call "SetDA.vi"("错误输入（无错误）"=w172, "DAVolt"=w161, "DANum"=u8 3, "DevIndex"=w173) -> ("错误输出"=w157:errorcluster, "DevIndex Output"=w158:i32)  [unwired: 6 in]
    n223 = case shown="真" "自动破膜" {
      tunnel: w147 -> [_ w411]
      frame False {
      }
      frame True {
        n224 = local read "Resistance"() -> (w410:dbl)
        n225 = Greater?(x=w410, y=800.0) -> (0:w412:bool)
        n226 = case shown="真" w412 {
          tunnel: w411 -> [_ w419]
          tunnel: w410 -> [_ w416]
          frame False {
            n227 = local write "自动破膜"(FALSE) -> ()
            n228 = One Button Dialog(message="没有达到GΩ封接，无法怕破膜" ("消息")) -> ()  [unwired: 1 in, 1 out]
          }
          frame True {
            n229 = Quotient & Remainder(x=w419, y=6) -> (x-y*floor(x/y)=w418:i32)  [unwired: 1 out]
            n230 = Not Equal?(x=w418, y=0) -> (x != y?=w417:bool)
            n231 = case shown="真" w417 {
              tunnel: w416 -> [w424 _]
              frame False {
                # "顿吸法，是否会损坏气箱"
                n232 = Greater?(x=w424, y=700.0) -> (0:w422:bool)
                n233 = case shown="真" w422 {
                  frame False {
                    n234 = local write "自动破膜"(FALSE) -> ()
                    n235 = One Button Dialog(message="破膜成功" ("消息")) -> ()  [unwired: 1 in, 1 out]
                  }
                  frame True {
                    w427 = FALSE
                    n236 = local write "大气压"(TRUE) -> ()
                    n237 = local write "高负开关"(FALSE) -> ()
                    n238 = local write "低负开关"(w427) -> ()
                    n239 = local write "高正开关"(w427) -> ()
                    n240 = local write "低正开关"(w427) -> ()
                  }
                }
              }
              frame True {
                n241 = flat-sequence {
                  frame #0 {
                    n242 = local write "高负"(-3.5) -> ()
                  }
                  frame #1 {
                    w431 = FALSE
                    w433 = FALSE
                    n243 = local write "高负开关"(TRUE) -> ()
                    n244 = local write "高负开关"(TRUE) -> ()
                    n245 = local write "低负开关"(w431) -> ()
                    n246 = local write "低负开关"(w433) -> ()
                    n247 = local write "大气压"(w431) -> ()
                    n248 = local write "大气压"(w433) -> ()
                    n249 = local write "低负开关"(w431) -> ()
                    n250 = local write "高正开关"(w431) -> ()
                  }
                }
              }
            }
          }
        }
      }
    }
    n251 = case shown="真" "入液阻值校准" {
      frame False {
      }
      frame True {
        n252 = flat-sequence {
          frame #0 {
            n253 = local read "阻值数组"() -> (w476:dbl[])
            n254 = Index Array(array=w476, index=9 ("索引")) -> (element=→"校准的入液阻值":dbl)
          }
          frame #1 {
            n255 = local write "入液阻值校准"(FALSE) -> ()
          }
        }
      }
    }
    n256 = property on="Image" class="ImageControl"() -> ("ROI"=w205:T12)  [unwired: 2 in, 2 out]
    n257 = Unbundle(w205) -> ("Global Rectangle"=w204:i32[])  [unwired: 1 out]
    n258 = Array Subset(array=w204, index=0 ("索引"), length=2 ("长度")) -> (w230:i32[])
    "目标坐标" <- w230
    n259 = local read "自动聚焦"() -> (w182:bool)
    n260 = local read "细调焦"() -> (w181:bool)
    n261 = Or(x=w182, y=w181) -> (x .or. y?=w183:bool)
    n262 = case shown="真" "自动移动" {
      tunnel: w232 -> [w814 w835]
      tunnel: [w814 w820] -> w209
      tunnel: w230 -> [_ w824]
      tunnel: w200 -> [_ w823]
      frame False {
      }
      frame True {
        # "模板针尖偏移量"
        # "PID控制针尖移动"
        # "可以直接用pid模块"
        n263 = Unbundle(w823) -> ("x"=w816:dbl, "x"=w822:dbl)
        n264 = Index Array(array=w824, index=1 ("索引")) -> (element=w833:i32)
        n265 = Subtract(x=w833, y=w822) -> (x-y=w829:dbl)
        n266 = Bundle("x"=w822, w833) -> ()  [unwired: 1 in, 1 out]
        n267 = Index Array(array=w824, index=0 ("索引")) -> (element=w834:i32)
        n268 = Add(x=sgl 0.0 ("y"), y=w816) -> (x+y=w815:dbl)
        n269 = Subtract(x=w834, y=w815) -> (x-y=w830:dbl)
        n270 = call-poly <vilib>:"PID.vi"("PID gains"="PID gains", "process variable"=w815, "setpoint"=w834) -> ("output"=w818:dbl)  [unwired: 7 in, 1 out]
        n271 = call-poly <vilib>:"PID.vi"("PID gains"="PID gains 2", "process variable"=w822, "setpoint"=w833) -> ("output"=w819:dbl)  [unwired: 7 in, 1 out]
        n272 = Bundle("x"=w816, w834) -> ()  [unwired: 1 in, 1 out]
        n273 = Square(x=w830) -> (x^2=w828:dbl)
        n274 = Square(x=w829) -> (x^2=w827:dbl)
        n275 = Add(x=w828, y=w827) -> (x+y=w821:dbl)
        n276 = Greater?(x=w821, y=10.0) -> (0:w836:bool)
        n277 = case shown="真" w836 {
          tunnel: w835 -> [w840 w844]
          tunnel: [w840 w843] -> w820
          tunnel: w818 -> [_ w842]
          tunnel: w819 -> [_ w841]
          frame False {
            n278 = local write "自动移动"(FALSE) -> ()
            n279 = One Button Dialog(message="针尖已移动到目标位置" ("消息")) -> ()  [unwired: 1 in, 1 out]
          }
          frame True {
            # "阈值范围需要调整，太大针尖检测不出来，太小程序会出现bug'"
            n280 = flat-sequence {
              tunnel: w844 -> [w851]
              tunnel: [w850] -> w843
              tunnel: w842 -> [w846]
              tunnel: w841 -> [w845]
              frame #0 {
                # "x位置p负号原因是设备转换后的"
                n281 = To Byte Integer(number=w845) -> (8bit integer=w849:i8)
                n282 = To Byte Integer(number=w846) -> (8bit integer=w848:i8)
                n283 = In Range and Coerce(upper limit=3.0 ("上限"), x=w849, lower limit=-3.0 ("上限")) -> (coerced(x)=w854:dbl)  [unwired: 1 out]
                n284 = In Range and Coerce(upper limit=3.0 ("上限"), x=w848, lower limit=-3.0 ("上限")) -> (coerced(x)=w847:dbl)  [unwired: 1 out]
                n285 = call "285A_RelMove.vi"("VISA资源名称"=w851, "Z 2"=0.0 ("Z"), "Y 2"=w854, "X 2"=w847) -> ("VISA resource name out 2"=w850:refnum<visa-resource-name>)  [unwired: 2 in, 5 out]
              }
            }
          }
        }
      }
    }
    n286 = case shown="真" w183 {
      tunnel: w237 -> [_ w394]
      tunnel: [0.0 ("Right") w393] -> w180
      tunnel: w233 -> [_ w392]
      tunnel: w199 -> [_ w391]
      frame False {
      }
      frame True {
        n287 = call "IMAQ Threshold"("Range"="Range", "Image Dst"=w394, "Image Src"=w391) -> ("Image Dst Out"=w381:T3)  [unwired: 7 in, 1 out]
        n288 = call "IMAQ LowPass"("Image Src"=w381) -> ("Image Dst Out"=w382:T3)  [unwired: 6 in, 1 out]
        n289 = call "IMAQ Copy"("Image Dst"=w392, "Image Src"=w382) -> ("Image Dst Out"=w389:T3)  [unwired: 4 in, 1 out]
        n290 = call "IMAQ RemoveParticle"("Number of Erosion"="Number of Erosion", "Image Src"=w389) -> ("Image Dst Out"=w383:T3)  [unwired: 8 in, 1 out]
        n291 = call "IMAQ Morphology"("Operation"="Operation", "Image Src"=w383) -> ("Image Dst Out"=w386:T3)  [unwired: 8 in, 1 out]
        n292 = call "IMAQ Convex Hull"("Image Src"=w386) -> ("Image Dst Out"=w387:T3)  [unwired: 9 in, 1 out]
        n293 = call "IMAQ FillHole"("Image Src"=w387) -> ("Image Dst Out"=w384:T3)  [unwired: 5 in, 1 out]
        n294 = call "IMAQ Clear Overlay"("Image"=w384) -> ("Image Out"=w380:T3)  [unwired: 9 in, 1 out]
        "二值化" <- w380
        n295 = call "IMAQ Particle Analysis Report"("Image"=w380) -> ("Particle Reports (Pixels)"=w379:T6)  [unwired: 5 in, 5 out]
        "Particle Reports (Pixels)" <- w379
        n296 = while {
          tunnel: w379 -> [w395]
          shift-right: [w404] -> w393
          shift-left: _ -> [w399]
          i -> [w397]
          stop <- w401 stop-if-true
          n297 = Equal?(x=w397, y=0) -> (x = y?=w398:bool)
          n298 = case shown="假" w398 {
            tunnel: w399 -> [w408 _]
            tunnel: [w408 0] -> w396
            frame False {
            }
            frame True {
            }
          }
          n299 = Index Array(array=w395, index=w397) -> (element=w406:T13)
          n300 = Unbundle(w406) -> ("Bounding Rect"=w407:T14)  [unwired: 5 out]
          n301 = Unbundle(w407) -> ("Right"=w402:dbl)  [unwired: 3 out]
          n302 = Equal?(x=w402, y=0.0) -> (x = y?=w401:bool)
          n303 = Greater?(x=w396, y=w402) -> (0:w405:bool)
          n304 = Select(t=w396, s=w405, f=w402) -> (s? t:f=w404:dbl)
        }
        "Right" <- w393
      }
    }
    "评价函数" <- w180
    n305 = case shown="5" "case" {
      tunnel: w158 -> [w268 w288 w310 w334 w358 w371]
      tunnel: w157 -> [w267 w287 w309 w333 w357 w370]
      tunnel: [w268 w270 w301 w328 w350 w368] -> w153
      tunnel: [w267 w278 w302 w327 w351 w367] -> w156
      tunnel: [w265 w269 w293 w317 w341 w365] -> w151
      frame Default {
        w266 = 0.0
        n306 = Bundle(w266, w266) -> (w265:cluster{dbl, dbl})  [unwired: 1 in]
      }
      frame 1 {
        w285 = TRUE
        w286 = FALSE
        n307 = Build Array(w286, w285, w285, w286, w286, w286, w286, w286) -> (w289:bool[])
        n308 = Boolean Array To Number(Boolean array=w289) -> (number=w292:u32)
        n309 = To Unsigned Byte Integer(number=w292) -> (unsigned 8bit integer=w291:u8)
        n310 = call "StartRead.vi"("错误输入（无错误）"=w287, "DevIndex"=w288) -> ("错误输出"=w283:errorcluster, "DevIndex Output"=w284:i32)  [unwired: 8 in]
        n311 = call "SetDioOut.vi"("错误输入（无错误）"=w283, "DioOut"=w291, "DioChanSel"=u8 255, "DevIndex"=w284) -> ("错误输出"=w279:errorcluster, "DevIndex Output"=w280:i32)  [unwired: 6 in]
        "错误输出 2" <- w279
        n312 = call "GetAiChans.vi"("错误输入（无错误）"=w279, "Num"=u32 1, "ChanSel"=u16 1, "DevIndex"=w280) -> ("错误输出"=w278:errorcluster, "Ai"=w275:sgl[][], "DevIndex Output"=w270:i32)  [unwired: 4 in, 1 out]
        n313 = Unbundle(w279) -> ()  [unwired: 3 out]
        n314 = Index Array(array=w275, index (row)=0, index (col)=0) -> (element=w272:sgl)
        n315 = local read "高正"() -> (w274:sgl)
        n316 = Multiply(x=w272, y=3) -> (x*y=w271:sgl)
        n317 = Bundle(w271, "高正"=w274) -> (w269:cluster{sgl, "高正":sgl})  [unwired: 1 in]
      }
      frame 2 {
        w308 = TRUE
        w307 = FALSE
        n318 = Build Array(w307, w308, w307, w307, w308, w307, w307, w307) -> (w311:bool[])
        n319 = Boolean Array To Number(Boolean array=w311) -> (number=w316:u32)
        n320 = To Unsigned Byte Integer(number=w316) -> (unsigned 8bit integer=w315:u8)
        n321 = call "StartRead.vi"("错误输入（无错误）"=w309, "DevIndex"=w310) -> ("错误输出"=w312:errorcluster, "DevIndex Output"=w313:i32)  [unwired: 8 in]
        n322 = call "SetDioOut.vi"("错误输入（无错误）"=w312, "DioOut"=w315, "DioChanSel"=u8 255, "DevIndex"=w313) -> ("错误输出"=w303:errorcluster, "DevIndex Output"=w304:i32)  [unwired: 6 in]
        n323 = call "GetAiChans.vi"("错误输入（无错误）"=w303, "Num"=u32 1, "ChanSel"=u16 2, "DevIndex"=w304) -> ("错误输出"=w302:errorcluster, "Ai"=w298:sgl[][], "DevIndex Output"=w301:i32)  [unwired: 4 in, 1 out]
        n324 = Unbundle(w303) -> ()  [unwired: 3 out]
        n325 = Index Array(array=w298, index (row)=0, index (col)=0) -> (element=w296:sgl)
        n326 = local read "高负"() -> (w297:sgl)
        n327 = Multiply(x=w296, y=-1.01) -> (x*y=w294:dbl)
        n328 = Bundle(w294, "高负"=w297) -> (w293:cluster{dbl, "高负":sgl})  [unwired: 1 in]
      }
      frame 3 {
        w319 = FALSE
        n329 = Build Array(w319, w319, w319, TRUE, w319, w319, w319, w319) -> (w335:bool[])
        n330 = Boolean Array To Number(Boolean array=w335) -> (number=w340:u32)
        n331 = To Unsigned Byte Integer(number=w340) -> (unsigned 8bit integer=w339:u8)
        n332 = call "StartRead.vi"("错误输入（无错误）"=w333, "DevIndex"=w334) -> ("错误输出"=w336:errorcluster, "DevIndex Output"=w337:i32)  [unwired: 8 in]
        n333 = call "SetDioOut.vi"("错误输入（无错误）"=w336, "DioOut"=w339, "DioChanSel"=u8 255, "DevIndex"=w337) -> ("错误输出"=w329:errorcluster, "DevIndex Output"=w330:i32)  [unwired: 6 in]
        n334 = call "GetAiChans.vi"("错误输入（无错误）"=w329, "Num"=u32 1, "ChanSel"=u16 4, "DevIndex"=w330) -> ("错误输出"=w327:errorcluster, "Ai"=w324:sgl[][], "DevIndex Output"=w328:i32)  [unwired: 4 in, 1 out]
        n335 = Unbundle(w329) -> ()  [unwired: 3 out]
        n336 = Index Array(array=w324, index (row)=0, index (col)=0) -> (element=w322:sgl)
        n337 = local read "低正"() -> (w323:sgl)
        n338 = Divide(x=w322, y=2.5) -> (x/y=w320:dbl)
        n339 = Bundle(w320, "低正"=w323) -> (w317:cluster{dbl, "低正":sgl})  [unwired: 1 in]
      }
      frame 4 {
        w342 = FALSE
        n340 = call "StartRead.vi"("错误输入（无错误）"=w357, "DevIndex"=w358) -> ("错误输出"=w360:errorcluster, "DevIndex Output"=w361:i32)  [unwired: 8 in]
        n341 = local read "低负"() -> (w346:sgl)
        n342 = Build Array(w342, w342, w342, w342, w342, TRUE, w342, w342) -> (w359:bool[])
        n343 = Boolean Array To Number(Boolean array=w359) -> (number=w364:u32)
        n344 = To Unsigned Byte Integer(number=w364) -> (unsigned 8bit integer=w363:u8)
        n345 = call "SetDioOut.vi"("错误输入（无错误）"=w360, "DioOut"=w363, "DioChanSel"=u8 255, "DevIndex"=w361) -> ("错误输出"=w352:errorcluster, "DevIndex Output"=w353:i32)  [unwired: 6 in]
        n346 = Unbundle(w352) -> ()  [unwired: 3 out]
        n347 = call "GetAiChans.vi"("错误输入（无错误）"=w352, "Num"=u32 1, "ChanSel"=u16 8, "DevIndex"=w353) -> ("错误输出"=w351:errorcluster, "Ai"=w347:sgl[][], "DevIndex Output"=w350:i32)  [unwired: 4 in, 1 out]
        n348 = Index Array(array=w347, index (row)=0, index (col)=0) -> (element=w345:sgl)
        n349 = Divide(x=w345, y=-2.299) -> (x/y=w343:dbl)
        n350 = Bundle(w343, "低负"=w346) -> (w341:cluster{dbl, "低负":sgl})  [unwired: 1 in]
      }
      frame 5 {
        w366 = 0.0
        (unwired) TRUE
        w369 = FALSE
        n351 = call "StartRead.vi"("错误输入（无错误）"=w370, "DevIndex"=w371) -> ("错误输出"=w373:errorcluster, "DevIndex Output"=w374:i32)  [unwired: 8 in]
        n352 = Build Array(w369, w369, w369, w369, w369, w369, w369, w369) -> (w372:bool[])
        n353 = Boolean Array To Number(Boolean array=w372) -> (number=w377:u32)
        n354 = To Unsigned Byte Integer(number=w377) -> (unsigned 8bit integer=w376:u8)
        n355 = call "SetDioOut.vi"("错误输入（无错误）"=w373, "DioOut"=w376, "DioChanSel"=u8 255, "DevIndex"=w374) -> ("错误输出"=w367:errorcluster, "DevIndex Output"=w368:i32)  [unwired: 6 in]
        n356 = Unbundle(w367) -> ()  [unwired: 3 out]
        n357 = Bundle(w366, w366) -> (w365:cluster{dbl, dbl})  [unwired: 1 in]
      }
    }
    "气压波形图表" <- w151
    n358 = case shown="真" "保存图像和数据" {
      tunnel: w199 -> [_ w573]
      tunnel: w209 -> [w546 w553]
      tunnel: [w546 w572] -> w194
      tunnel: w208 -> [_ w571]
      tunnel: w147 -> [_ w566]
      tunnel: w207 -> [_ w552]
      tunnel: w179 -> [w545 w548]
      tunnel: [w545 w547] -> w178
      frame False {
      }
      frame True {
        w555 = "\t"
        # "数据记录"
        n359 = disable-structure shown="禁用" {
          frame Disabled {
            n360 = call "285A_RelMove.vi"("Z 2"=2.0 ("Y 2"), "Y 2"=0.0, "X 2"=0.0) -> ()  [unwired: 3 in, 6 out]
          }
          frame Enabled {
          }
        }
        n361 = call "285A_GetPos.vi"("VISA资源名称"=w553) -> ("Z"=w567:dbl, "Y"=w568:dbl, "X"=w569:dbl, "VISA资源名称输出"=w572:refnum<visa-resource-name>)  [unwired: 5 in, 2 out]
        n362 = Number To Fractional String(number=w569) -> (F-format string=w560:string)  [unwired: 3 in]
        n363 = Number To Fractional String(number=w568) -> (F-format string=w558:string)  [unwired: 3 in]
        n364 = Number To Fractional String(number=w567) -> (F-format string=w556:string)  [unwired: 3 in]
        n365 = Number To Decimal String(number=w566) -> (decimal integer string=w549:string)  [unwired: 1 in]
        n366 = Number To Fractional String(number=w571) -> (F-format string=w551:string)  [unwired: 3 in]
        n367 = Concatenate Strings(w549, w555, "X轴：" ("字符串"), w560, w555, "Y轴：" ("字符串"), w558, w555, "Z轴：" ("字符串"), w556, w555, "阻值：" ("字符串"), w551, "\n") -> (w570:string)
        n368 = Concatenate Strings("图像" ("字符串"), w549, ".jpg" ("字符串")) -> (w565:string)
        n369 = Build Path(base path=w552, name or relative path=w565) -> (appended path=w562:path)
        n370 = Write to Text File(file (use dialog)=w548, text=w570) -> (refnum out=w547:refnum<file>)  [unwired: 2 in, 2 out]
        n371 = call-poly "IMAQ Write File 2"("File Path"=w562, "Image"=w573) -> ()  [unwired: 8 in, 2 out]
      }
    }
    n372 = Tick Count (ms)() -> (millisecond timer value=w188:u32)
    n373 = Subtract(x=w188, y=w189) -> (x-y=→"循环时间":u32)
    n374 = case shown="真" "自动封接" {
      frame False {
        "封接负压增幅" <- 0.0
      }
      frame True {
        w439 = 1000.0 ("y")
        # "斜率负压法"
        # "自动根据阻值改变气压"
        n375 = local read "阻值数组"() -> (w450:dbl[])
        n376 = Index Array(array=w450, index=0 ("索引")) -> (element=w438:dbl)
        n377 = Index Array(array=w450, index=1 ("索引")) -> (element=w437:dbl)
        n378 = Index Array(array=w450, index=2 ("索引")) -> (element=w452:dbl)
        n379 = Index Array(array=w450, index=3 ("索引")) -> (element=w451:dbl)
        n380 = Index Array(array=w450, index=4 ("索引")) -> (element=w449:dbl)
        n381 = Greater?(x=w438, y=w439) -> (0:w448:bool)
        n382 = Greater?(x=w452, y=w439) -> (0:w445:bool)
        n383 = Greater?(x=w437, y=w439) -> (0:w447:bool)
        n384 = Greater?(x=w451, y=w439) -> (0:w443:bool)
        n385 = Greater?(x=w449, y=w439) -> (0:w441:bool)
        n386 = And(x=w448, y=w447) -> (x .and. y?=w446:bool)
        n387 = And(x=w446, y=w445) -> (x .and. y?=w444:bool)
        n388 = And(x=w444, y=w443) -> (x .and. y?=w442:bool)
        n389 = And(x=w442, y=w441) -> (x .and. y?=w440:bool)
        n390 = Subtract(x=w438, y=w437) -> (x-y=w436:dbl)
        n391 = case shown="真" w440 {
          tunnel: w436 -> [w460 _]
          frame False {
            n392 = flat-sequence {
              tunnel: w458 -> [w466]
              frame #0 {
                n393 = local read "封接负压增幅"() -> (w461:dbl)
                n394 = Add(x=-1.0, y=w461) -> (x+y=w462:dbl)
                n395 = local write "低负"(w462) -> ()
              }
              frame #1 {
                w464 = FALSE
                n396 = local write "低负开关"(TRUE) -> ()
                n397 = local write "高正开关"(w464) -> ()
                n398 = local write "高负开关"(w464) -> ()
                n399 = local write "低正开关"(w464) -> ()
                n400 = local write "大气压"(w464) -> ()
              }
              frame #2 {
                n401 = case shown="真" w466 {
                  frame False {
                    n402 = local read "封接负压增幅"() -> (w469:dbl)
                    n403 = Add(x=w469, y=-0.1) -> (x+y=w467:dbl)
                    n404 = local write "封接负压增幅"(w467) -> ()
                  }
                  frame True {
                    n405 = local read "封接负压增幅"() -> (w472:dbl)
                    n406 = Add(x=w472, y=0.1) -> (x+y=w470:dbl)
                    n407 = local write "封接负压增幅"(w470) -> ()
                  }
                }
              }
            }
            n408 = Greater?(x=w460, y=10.0) -> (0:w458:bool)
          }
          frame True {
            n409 = local write "自动封接"(FALSE) -> ()
          }
        }
      }
    }
    n410 = Unbundle(w151) -> (→"测量值":dbl, "高正"=→"给定值":dbl)
    n411 = case shown="真" "自动接触" {
      tunnel: w194 -> [w520 w529]
      tunnel: [w520 w528] -> w193
      frame False {
      }
      frame True {
        # "阈值"
        n412 = local read "校准的入液阻值"() -> (w526:dbl)
        n413 = local read "阻值数组"() -> (w535:dbl[])
        n414 = Index Array(array=w535, index=0 ("索引")) -> (element=w527:dbl)
        n415 = Index Array(array=w535, index=1 ("索引")) -> (element=w533:dbl)
        n416 = Index Array(array=w535, index=2 ("索引")) -> (element=w532:dbl)
        n417 = Add(x=0.25, y=w526) -> (x+y=w524:dbl)
        n418 = Greater?(x=w527, y=w533) -> (0:w531:bool)
        n419 = Greater?(x=w533, y=w532) -> (0:w530:bool)
        n420 = Greater?(x=w527, y=w524) -> (0:w523:bool)
        n421 = And(x=w531, y=w530) -> (x .and. y?=w522:bool)
        n422 = And(x=w523, y=w522) -> (x .and. y?=w521:bool)
        n423 = case shown="假" w521 {
          tunnel: w529 -> [w541 w543]
          tunnel: [w542 w543] -> w528
          frame False {
            # "向下运动"
            n424 = call "285A_RelMove.vi"("VISA资源名称"=w541, "Z 2"="下降步伐/um", "Y 2"=0.0, "X 2"=0.0) -> ("VISA resource name out 2"=w542:refnum<visa-resource-name>)  [unwired: 2 in, 5 out]
          }
          frame True {
            n425 = local write "自动接触"(FALSE) -> ()
          }
        }
      }
    }
    n426 = event shown="[4] \"低负开关\": 值改变" {
      selector: _ -> [_ _ _ _ _ _]
      dyn-events: _ -> [_ _ _ _ _ _]
      timeout: 10 -> [_ _ _ _ _ _]
      event "高正开关": Value Change {
        n427 = event-data() -> ("OldVal"=w245:bool)  [unwired: 1 in, 5 out]
        n428 = local read "高正开关"() -> (w246:bool)
        n429 = case shown="假" w246 {
          tunnel: w245 -> [_ w248]
          frame False {
          }
          frame True {
            n430 = local write "高负开关"(w248) -> ()
            n431 = local write "低负开关"(w248) -> ()
            n432 = local write "低正开关"(w248) -> ()
            n433 = local write "大气压"(w248) -> ()
            n434 = local write "case"(1.0) -> ()
          }
        }
      }
      event Timeout {
        n435 = event-data() -> ()  [unwired: 1 in, 3 out]
      }
      event "大气压": Value Change {
        n436 = event-data() -> ("OldVal"=w249:bool)  [unwired: 1 in, 5 out]
        n437 = local read "大气压"() -> (w250:bool)
        n438 = case shown="假" w250 {
          tunnel: w249 -> [_ w252]
          frame False {
          }
          frame True {
            n439 = local write "高负开关"(w252) -> ()
            n440 = local write "低正开关"(w252) -> ()
            n441 = local write "低负开关"(w252) -> ()
            n442 = local write "高正开关"(w252) -> ()
            n443 = local write "case"(5.0) -> ()
          }
        }
      }
      event "低正开关": Value Change {
        n444 = event-data() -> ("OldVal"=w254:bool)  [unwired: 1 in, 5 out]
        n445 = local read "低正开关"() -> (w253:bool)
        n446 = case shown="真" w253 {
          tunnel: w254 -> [_ w256]
          frame False {
          }
          frame True {
            n447 = local write "高正开关"(w256) -> ()
            n448 = local write "高负开关"(w256) -> ()
            n449 = local write "低负开关"(w256) -> ()
            n450 = local write "大气压"(w256) -> ()
            n451 = local write "case"(3.0) -> ()
          }
        }
      }
      event "低负开关": Value Change {
        n452 = event-data() -> ("OldVal"=w258:bool)  [unwired: 1 in, 5 out]
        n453 = local read "低负开关"() -> (w257:bool)
        n454 = case shown="真" w257 {
          tunnel: w258 -> [_ w260]
          frame False {
          }
          frame True {
            n455 = local write "高负开关"(w260) -> ()
            n456 = local write "低正开关"(w260) -> ()
            n457 = local write "高正开关"(w260) -> ()
            n458 = local write "大气压"(w260) -> ()
            n459 = local write "case"(4.0) -> ()
          }
        }
      }
      event "高负开关": Value Change {
        n460 = event-data() -> ("OldVal"=w262:bool)  [unwired: 1 in, 5 out]
        n461 = local read "高负开关"() -> (w261:bool)
        n462 = case shown="真" w261 {
          tunnel: w262 -> [_ w264]
          frame False {
          }
          frame True {
            n463 = local write "低正开关"(w264) -> ()
            n464 = local write "低负开关"(w264) -> ()
            n465 = local write "高正开关"(w264) -> ()
            n466 = local write "大气压"(w264) -> ()
            n467 = local write "case"(2.0) -> ()
          }
        }
      }
    }
    n468 = Wait (ms)(milliseconds to wait=u32 1 ("毫秒计时值")) -> ()  [unwired: 1 out]
  }
  n469 = One Button Dialog(message="准备工作是否完成：  \n1设备是否都打开      \n2微电极是否装配      \n3气动箱是否调试      \n4电极银丝是否合格   \n5细胞是否准备完好   \n6参比电极是否插入液\n" ("消息")) -> ()  [unwired: 1 in, 1 out]
  n470 = disable-structure shown="禁用" {
    frame Disabled {
      n471 = call "285A_Move.vi"("Abso_Z"=0.0, "Abso_Y"=0.0, "Abso_X"=0.0) -> ()  [unwired: 5 in, 4 out]
      n472 = call "AI0.vi"() -> ()  [unwired: 10 in, 2 out]
      n473 = call "285A_SetVelRes_velres.vi"() -> ()  [unwired: 11 in, 1 out]
      n474 = call "285A_GetPos.vi"() -> ()  [unwired: 6 in, 6 out]
    }
    frame Enabled {
    }
  }
  n475 = Close File(refnum=w51) -> ()  [unwired: 1 in, 2 out]
  n476 = call "285A_Update.vi"("VISA资源名称"=w84) -> ("VISA资源名称 2"=w83:refnum<visa-resource-name>)  [unwired: 9 in, 1 out]
  n477 = call "Imaq Dispose"("Image"=w97) -> ()  [unwired: 5 in, 1 out]
  n478 = call <vilib>:"IMAQdx Close Camera.vi"("error in"=w98, "Session In"=w96) -> ("error out"=w99:errorcluster)  [unwired: 9 in]
  n479 = call "SetDA.vi"("错误输入（无错误）"=w2, "DANum"=w3) -> ("错误输出"=w23:errorcluster, "DevIndex Output"=w24:i32)  [unwired: 8 in]
  n480 = VISA Close(VISA resource name=w83) -> ()  [unwired: 1 in, 1 out]
  n481 = call "SetDA.vi"("错误输入（无错误）"=w23, "DAVolt"=0.0, "DANum"=u8 1, "DevIndex"=w24) -> ("错误输出"=w22:errorcluster, "DevIndex Output"=w21:i32)  [unwired: 6 in]
  n482 = Build Array(w12, w12, w12, w12, w12, w12, w12, w12) -> (w10:bool[])
  n483 = call "SetDA.vi"("错误输入（无错误）"=w22, "DAVolt"=0.0, "DANum"=u8 2, "DevIndex"=w21) -> ("错误输出"=w19:errorcluster, "DevIndex Output"=w20:i32)  [unwired: 6 in]
  n484 = Boolean Array To Number(Boolean array=w10) -> (number=w11:u32)
  n485 = call "SetDA.vi"("错误输入（无错误）"=w19, "DAVolt"=0.0, "DANum"=u8 3, "DevIndex"=w20) -> ("错误输出"=w6:errorcluster, "DevIndex Output"=w7:i32)  [unwired: 6 in]
  n486 = To Unsigned Byte Integer(number=w11) -> (unsigned 8bit integer=w9:u8)
  n487 = call "SetDioOut.vi"("错误输入（无错误）"=w6, "DioOut"=w9, "DioChanSel"=u8 255, "DevIndex"=w7) -> ("错误输出"=w5:errorcluster, "DevIndex Output"=w4:i32)  [unwired: 6 in]
  n488 = call "StopRead.vi"("错误输入（无错误）"=w5, "DevIndex"=w4) -> ("错误输出"=w30:errorcluster, "DevIndex Output"=w31:i32)  [unwired: 8 in]
  n489 = call "SetSoftTrig.vi"("错误输入（无错误）"=w30, "Trig"=u8 0, "DevIndex"=w31) -> ("错误输出"=w29:errorcluster, "DevIndex Output"=w27:i32)  [unwired: 7 in]
  n490 = call "ClearTrigger.vi"("错误输入（无错误）"=w29, "DevIndex"=w27) -> ("错误输出"=w28:errorcluster, "DevIndex Output"=w26:i32)  [unwired: 8 in]
  n491 = call "ClearBufs.vi"("错误输入（无错误）"=w28, "DevIndex"=w26) -> ("错误输出"=w32:errorcluster, "DevIndex Output"=w33:i32)  [unwired: 8 in]
  n492 = call "CloseDevice.vi"("错误输入（无错误）"=w32, "DevIndex"=w33) -> ("错误输出"=w1:errorcluster)  [unwired: 8 in, 1 out]
  n493 = Merge Errors(w79, w1) -> (w80:errorcluster)
  n494 = Merge Errors(w99, w80) -> (→"错误输出":errorcluster)
